vi "Sort XYZ piezos metadata.vi"(0 "reference in":refnum<class "metadata.lvclass">, 5 "error in (no error)":errorcluster) -> (14 "reference out":refnum<class "metadata.lvclass">, 16 "XYZ piezos":T1, 19 "error out":errorcluster)   [LabVIEW 2019, in "metadata.lvclass"]
uses:
  metadata.lvclass
  XYZ piezos parameters.ctl
  Error not found -- string property value.ctl
panel:
  out "Array":string[](array[string])
  out "Array 2":i32[](array[numeric])
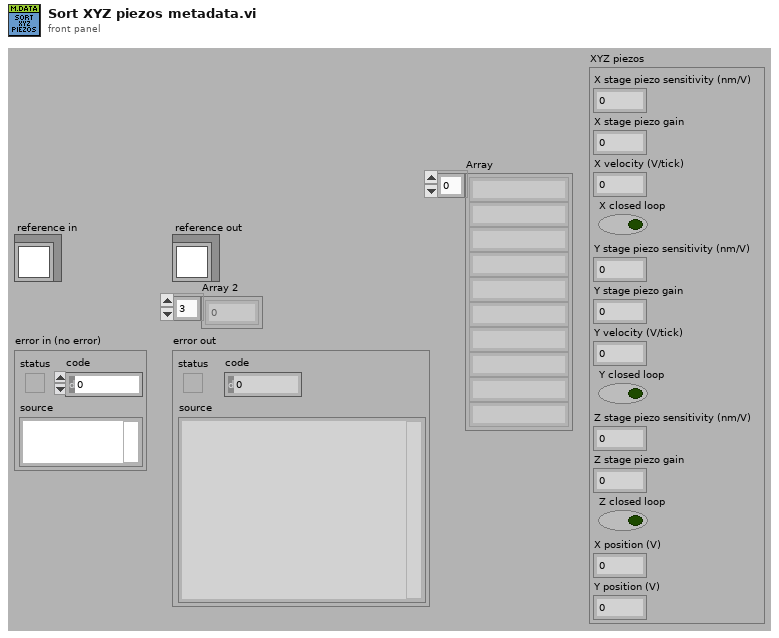
[diagram p1: front panel]
types:
  T1 = typedef "metadata.lvclass/XYZ piezos parameters.ctl" = cluster{"X stage piezo sensitivity (nm/V)":dbl, "X stage piezo gain":dbl, "X velocity (V/tick)":dbl, "X closed loop":bool, "Y stage piezo sensitivity (nm/V)":dbl, "Y stage piezo gain":dbl, "Y velocity (V/tick)":dbl, "Y closed loop":bool, "Z stage piezo sensitivity (nm/V)":dbl, "Z stage piezo gain":dbl, "Z closed loop":bool, "X position (V)":dbl, "Y position (V)":dbl}
  T2 = typedef "metadata.lvclass/Error not found -- string property value.ctl" = string
  T3 = typedef "metadata.lvclass/ObjectAttributesRef.ctl" = refnum<data-value>
  T4 = typedef "metadata.lvclass/ObjectAttributes.ctl" = cluster{"MyAttribute":dbl, "System Control":T5, "file info":T6, "Sample info":T7, "Cantilever info":T8, "XYZ piezos":T1, "Mapping":T9, "Fcurve segment":T10[], "Fast fpga segment":T12, "Chirp":T13, "precision (6)":i16, "width (-)":i16, "Metadata":T14, "config filepath":path, "Section names []":string[], "Property names []":string[], "nb elements":u16}
  T5 = typedef "metadata.lvclass/System control parameters.ctl" = cluster{"FPGA SW version":string, "TDMS file version":string, "Instrument":string, "Instrument model":string, "Instrument scanner":string, "Instrument clockrate (Mhz)":string, "Instrument tick time (us)":string}
  T6 = typedef "metadata.lvclass/File info parameters.ctl" = cluster{"Time Stamp":timestamp, "Filename":string, "Filepath":path, "User":string, "Experiment_name":string, "Curve_id":string, "number_segments":u8, "number_consecutive_scans":u32}
  T7 = typedef "metadata.lvclass/Sample info parameters.ctl" = cluster{"Sample name":string, "Sample species":string}
  T8 = typedef "metadata.lvclass/Cantilever info parameters.ctl" = cluster{"spring constant calib method":string, "invOLS calib method":string, "thermal calib deflection channel":string, "model":string, "shape":string, "tip geometry":string, "Laser sum (V)":dbl, "Laser power (mA)":dbl, "invOLS_(nm/V)":dbl, "spring constant nominal (N/m)":dbl, "spring constant calib (N/m)":dbl, "resosnance frequency air calib (Hz)":dbl, "resosnance frequency calib (Hz)":dbl, "quality factor":dbl, "Acoefficident_GCI_(nN.s^1.3/m)":dbl, "half angle (deg)":dbl, "tip radius (m)":dbl, "tip height (m)":dbl, "system mount angle (deg)":dbl}
  T9 = typedef "metadata.lvclass/Mapping parameters.ctl" = cluster{"Mapping":bool, "index":u16, "position row":u16, "position column":u16, "next position row":i16, "next position column":i16, "X initial position (V)":dbl, "Y initial position (V)":dbl, "X step size (V)":dbl, "Y step size (V)":dbl}
  T10 = typedef "metadata.lvclass/Fcurve segment.ctl" = cluster{"type":T11, "fast_fpga_trigger":bool, "nb":u8, "duration (ticks)":i64, "nb points":i32, "sampling rate (S/s)":u32, "Zpiezo control out":string, "initial deflection (V)":dbl, "relative setpoint":bool, "setpoint on":bool, "setpoint (V)":dbl, "setpoint trigger channel":string, "velocity (V/tick)":dbl, "Z position setpoint trigger (V)":dbl, "Z retract length (V)":dbl, "dec factor":u32}
  T11 = typedef "metadata.lvclass/Segment type--combobox.ctl" = string
  T12 = typedef "metadata.lvclass/fast fpga segment parameters.ctl" = cluster{"Fast start time trigger":timestamp, "nb_points":u32, "sampling_rate_(S/s)":u32, "duration_(ticks)":u32}
  T13 = typedef "metadata.lvclass/Chirp added parameters.ctl" = cluster{"f start (Hz)":dbl, "f end (Hz)":dbl, "Sweep type":string}
  T14 = typedef "metadata.lvclass/Metadata output --cluster.ctl" = cluster{"Property Names":string[], "Property Values":variant[]}
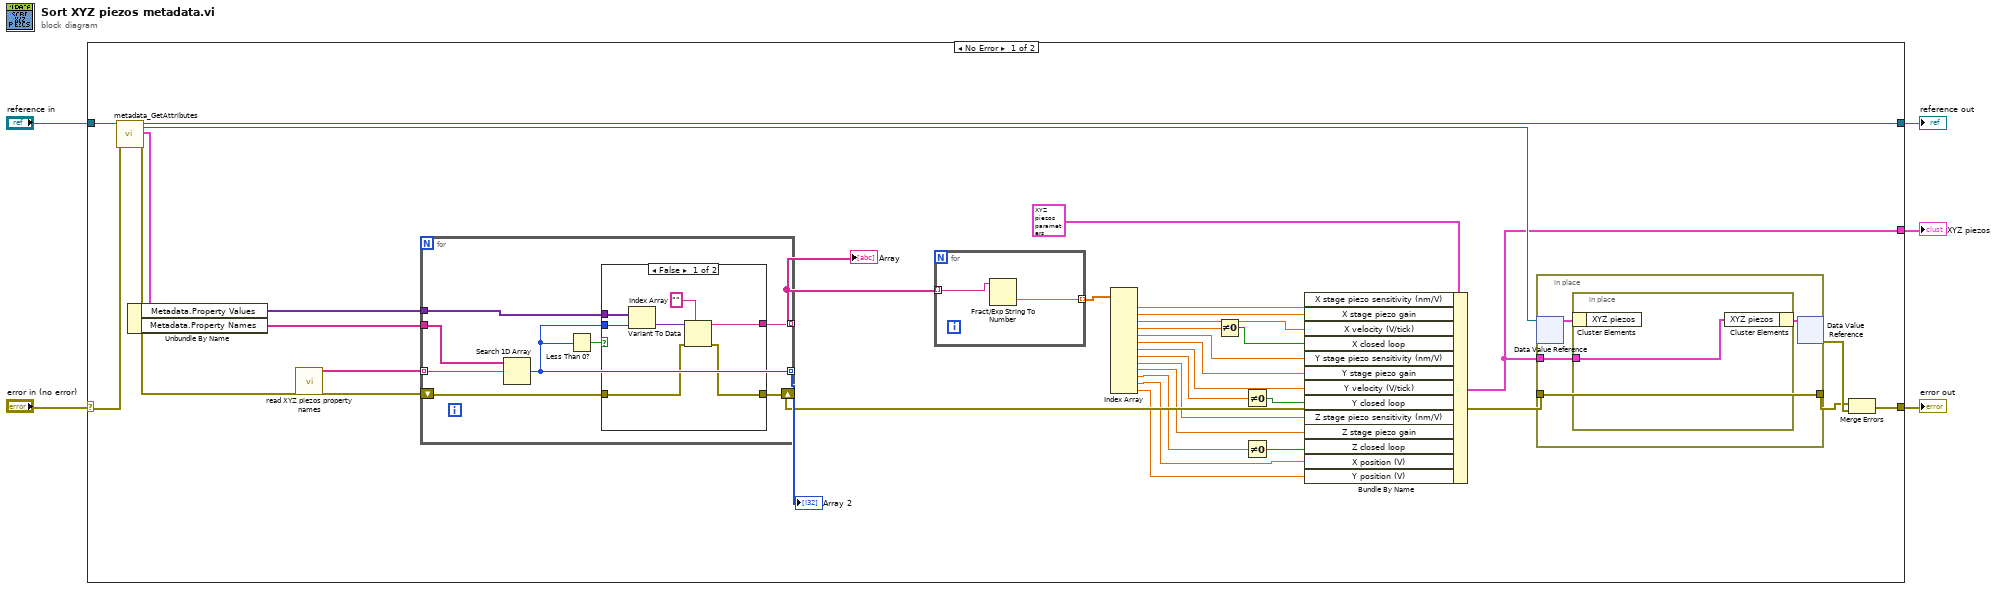
[diagram p0: block diagram]
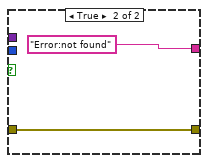
[diagram p2: hidden frame]
diagram:
  n1 = case shown="No Error" "error in (no error)" {
    selector: "error in (no error)" -> [w36 w66]
    tunnel: [w40 w66] -> w4
    tunnel: [w35 w65] -> w2
    tunnel: "reference in" -> [w37 w65]
    tunnel: [w28 _] -> w1
    frame No Error {
      n2 = call "metadata_GetAttributes.vi"("reference in"=w37, "error in (no error)"=w36) -> ("reference out"=w35:refnum<class "metadata.lvclass">, "attributes ref"=w34:T3, "attributes"=w33:T4, "error out"=w27:errorcluster)  [unwired: 14 in]
      n3 = Unbundle By Name(w33) -> ("Metadata.Property Values"=w29:variant[], "Metadata.Property Names"=w32:string[])
      n4 = call "read XYZ piezos property names.vi"("error in (no error)"=w27) -> ("XYZ piezos"=w25:string[], "error out"=w26:errorcluster)  [unwired: 17 in]
      n5 = for {
        tunnel: w25 -> [w50] mode=indexing
        tunnel: [w44] -> w31 mode=indexing
        shift-right: [w45] -> w30
        shift-left: w26 -> [w46]
        tunnel: w32 -> [w49]
        tunnel: w29 -> [w48]
        tunnel: [w47] -> w6 mode=indexing
        n6 = Search 1D Array(1D array=w49, element=w50) -> (index of element=w44:i32)  [unwired: 1 in]
        n7 = Less Than 0?(x=w44) -> (x < 0?=w43:bool)
        n8 = case shown="False" w43 {
          tunnel: w48 -> [w57 _]
          tunnel: w44 -> [w56 _]
          tunnel: [w54 T2 "Error:not found" ("Error")] -> w47
          tunnel: w46 -> [w53 w59]
          tunnel: [w52 w59] -> w45
          frame False {
            n9 = Index Array(array=w57, index=w56) -> (element=w55:variant)
            n10 = Variant To Data(error in=w53, type="", Variant=w55) -> (data=w54:string, error out=w52:errorcluster)
          }
          frame True {
          }
        }
      }
      "Array 2" <- w31
      "Array" <- w6
      n11 = for {
        tunnel: [w42] -> w23 mode=indexing
        tunnel: w6 -> [w41] mode=indexing
        n12 = Fract/Exp String To Number(string=w41) -> (number=w42:dbl)  [unwired: 3 in, 1 out]
      }
      n13 = Index Array(array=w23) -> (element #1=w22:dbl, element #2=w21:dbl, element #3=w20:dbl, element #4=w19:dbl, element #5=w17:dbl, element #6=w16:dbl, element #7=w15:dbl, element #8=w14:dbl, element #9=w12:dbl, element #10=w11:dbl, element #11=w10:dbl, element #12=w8:dbl, element #13=w7:dbl)  [unwired: 13 in]
      n14 = Not Equal To 0?(x=w19) -> (x != 0?=w18:bool)
      n15 = Not Equal To 0?(x=w14) -> (x != 0?=w13:bool)
      n16 = Not Equal To 0?(x=w10) -> (x != 0?=w9:bool)
      n17 = Bundle By Name(cluster=T1 {"X stage piezo sensitivity (nm/V)"=0.0, "X stage piezo gain"=0.0, "X velocity (V/tick)"=0.0, "X closed loop"=FALSE, "Y stage piezo sensitivity (nm/V)"=0.0, "Y stage piezo gain"=0.0, "Y velocity (V/tick)"=0.0, "Y closed loop"=FALSE, "Z stage piezo sensitivity (nm/V)"=0.0, "Z stage piezo gain"=0.0, "Z closed loop"=FALSE, "X position (V)"=0.0, "Y position (V)"=0.0} ("XYZ piezos"), "X stage piezo sensitivity (nm/V)"=w22, "X stage piezo gain"=w21, "X velocity (V/tick)"=w20, "X closed loop"=w18, "Y stage piezo sensitivity (nm/V)"=w17, "Y stage piezo gain"=w16, "Y velocity (V/tick)"=w15, "Y closed loop"=w13, "Z stage piezo sensitivity (nm/V)"=w12, "Z stage piezo gain"=w11, "Z closed loop"=w9, "X position (V)"=w8, "Y position (V)"=w7) -> (w28:T1)
      n18 = in-place {
        in-place-border: w30 -> [w61]
        in-place-border: [w61] -> w38
        in-place-border: w28 -> [w60]
        n19 = in-place-dvr #1(w34) -> (w62:T4)  [unwired: 1 out]
        n20 = in-place {
          in-place-border: w60 -> [w64]
          n21 = in-place-cluster #2(w62) -> ()  [unwired: 1 out]
          n22 = in-place-cluster #2("XYZ piezos"=w64) -> (w63:T4)
        }
        n23 = in-place-dvr #1(w63) -> (w39:errorcluster)  [unwired: 1 out]
      }
      n24 = Merge Errors(w38, w39) -> (w40:errorcluster)
    }
    frame Error {
    }
  }
  "error out" <- w4
  "reference out" <- w2
  "XYZ piezos" <- w1
